vi "Setup.vi"(9 "Active Project":refnum<vi>, 10 "NI.LV.Dialog Instance":refnum<vi>) -> (1 "Project Type Name Library File Path":T1, 2 "Target":string, 3 "Project Stuff out":refnum<class "Project Stuff.lvclass">, 4 "All Type Name Library File Path":T1)   [LabVIEW 2020, in "_Shared.lvlib" / "Project Stuff.lvclass"]
uses:
  Project Stuff.lvclass
  Project Stuff.lvclass/Project Stuff.ctl
  <vilib>/Utility/EditLVProj/Edit LVProj.lvlib
  Refs.ctl
  Library.ctl
  VI.ctl
  _Shared.lvlib
  Name Library File Path.ctl
  Type.ctl
  Type Name Library File Path.ctl
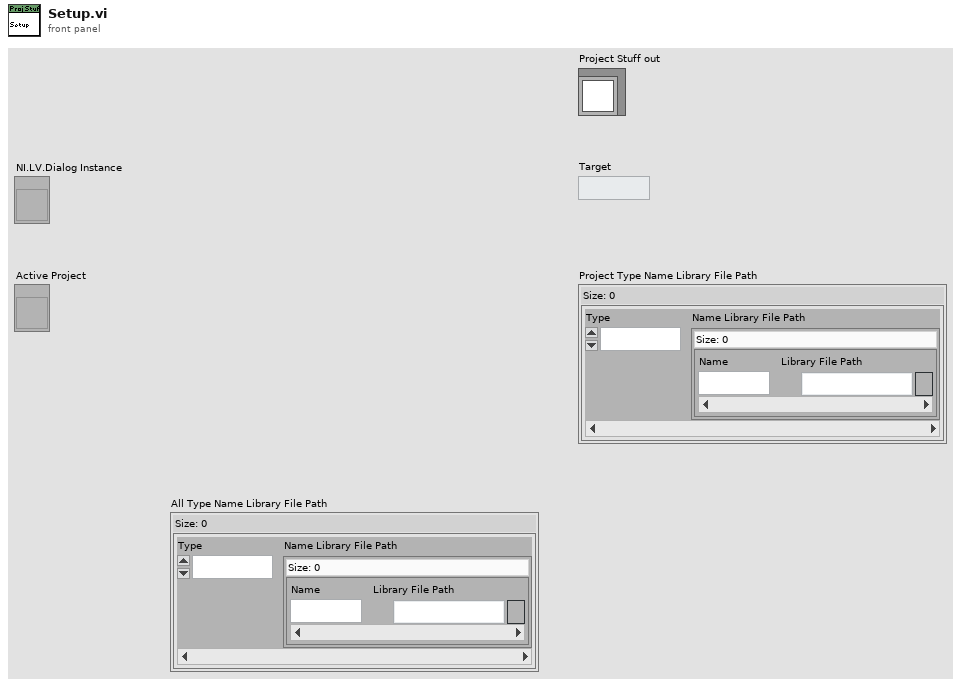
[diagram p1: front panel]
types:
  T1 = typedef "_Shared.lvlib/Type Name Library File Path.ctl" = map{T2, T3}
  T2 = typedef "_Shared.lvlib/Type.ctl" = enum16{"Actor", "Msg"}
  T3 = typedef "_Shared.lvlib/Name Library File Path.ctl" = map{string, path}
  T4 = typedef "_Shared.lvlib/Project Stuff.lvclass/Library.ctl" = set{refnum<vi>}
  T5 = typedef "_Shared.lvlib/Project Stuff.lvclass/VI.ctl" = set{refnum<vi>}
  T6 = typedef "_Shared.lvlib/Project Stuff.lvclass/Refs.ctl" = cluster{"Target":refnum<vi>, "VI":T5, "Library":T4}
  T7 = typedef "Edit LVProj.lvlib/Library And VI References.ctl" = cluster{"Target Reference":refnum<vi>, "VI References":refnum<vi>[], "Library References":refnum<vi>[]}
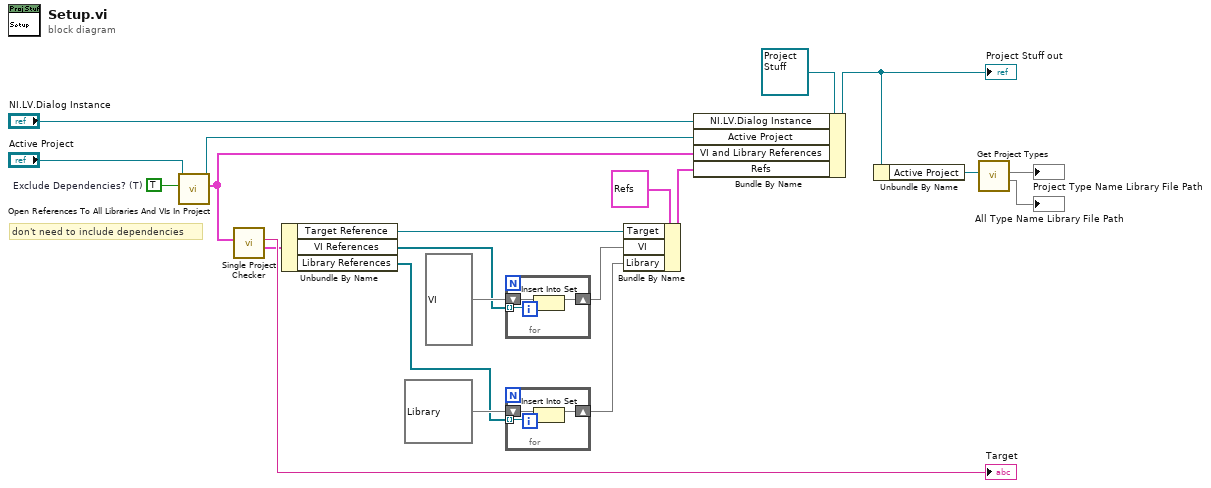
[diagram p0: block diagram]
diagram:
  w20 = TRUE  # Exclude Dependencies? (T)
  # "don't need to include dependencies"
  n1 = call <vilib>:"Open References To All Libraries And VIs In Project.vi"("Exclude Dependencies? (T)"=w20, "Project in"="Active Project") -> ("VI and Library References"=w5:T7[], "Project out"=w21:refnum<vi>)  [unwired: 7 in, 1 out]
  n2 = call "Single Project Checker.vi"("VI and Library References"=w5) -> ("Ref"=w9:T7, "Target"=→"Target":string)  [unwired: 9 in]
  n3 = Unbundle By Name(w9) -> ("Target Reference"=w8:refnum<vi>, "VI References"=w12:refnum<vi>[], "Library References"=w10:refnum<vi>[])
  n4 = for {
    shift-right: [w23] -> w7
    shift-left: T5 {} ("VI") -> [w24]
    tunnel: w12 -> [w22] mode=indexing
    n5 = Insert Into Set(10:w22, 11:w24) -> (3:w23:T5)  [unwired: 1 out]
  }
  n6 = for {
    shift-right: [w26] -> w6
    shift-left: T4 {} ("Library") -> [w27]
    tunnel: w10 -> [w25] mode=indexing
    n7 = Insert Into Set(10:w25, 11:w27) -> (3:w26:T4)  [unwired: 1 out]
  }
  n8 = Bundle By Name(cluster=T6 {"Target"=refnum, "VI"={}, "Library"={}} ("Refs"), "Target"=w8, "VI"=w7, "Library"=w6) -> (w14:T6)
  n9 = Bundle By Name(cluster=refnum<class "Project Stuff.lvclass"> refnum ("Project Stuff out"), "NI.LV.Dialog Instance"="NI.LV.Dialog Instance", "Active Project"=w21, "VI and Library References"=w5, "Refs"=w14) -> (w4:refnum<class "Project Stuff.lvclass">)
  "Project Stuff out" <- w4
  n10 = Unbundle By Name(w4) -> ("Active Project"=w3:refnum<vi>)
  n11 = call "Get Project Types.vi"("Project:Active Project"=w3) -> ("All Type Name Library File Path"=→"All Type Name Library File Path":T1, "Project Type Name Library File Path"=→"Project Type Name Library File Path":T1)  [unwired: 9 in]
